vi "Begin Mouse.vi"(3 "Mouse IO":T1) -> (1 "Mouse IO out":T1)   [LabVIEW 2012]
uses:
  <vilib>/eio/EIONode/EIONode.xnode
  <vilib>/rvi/eio/common/nirviEmuTemplateMethod_errors.vi
  <vilib>/eio/EIOMethodNode/EIOMethodNode.xnode
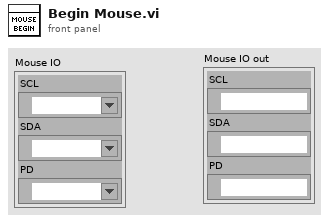
[diagram p1: front panel]
types:
  T1 = cluster{"SCL":refnum<k21>, "SDA":refnum<k21>, "PD":refnum<k21>}
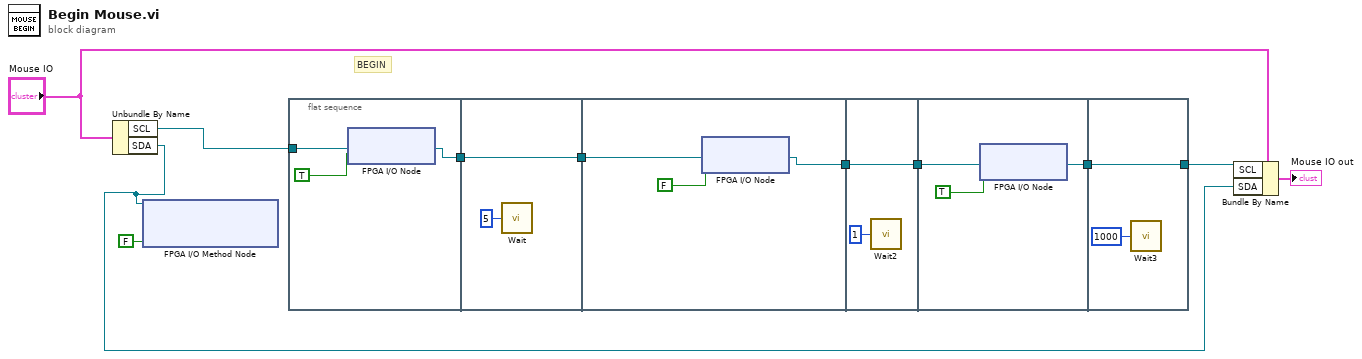
[diagram p0: block diagram]
diagram:
  # "BEGIN"
  n1 = Unbundle By Name("Mouse IO") -> ("SCL"=w7:refnum<k21>, "SDA"=w2:refnum<k21>)
  n2 = xnode "FPGA I/O Method Node"("FPGA I/O In"=w2, "Enable"=FALSE) -> ()  [unwired: 1 out]
  n3 = flat-sequence {
    tunnel: w7 -> [w14]
    tunnel: [w12] -> w11
    tunnel: [w16] -> w10
    tunnel: w11 -> [w16]
    tunnel: w10 -> [w18]
    tunnel: [w17] -> w9
    tunnel: [w21] -> w8
    tunnel: w9 -> [w21]
    tunnel: w8 -> [w23]
    tunnel: [w22] -> w5
    tunnel: [w25] -> w4
    tunnel: w5 -> [w25]
    frame #0 {
      n4 = xnode "FPGA I/O Node"("I/O Item"=TRUE, "FPGA I/O In"=w14) -> ("FPGA I/O Out"=w12:refnum<k21>)
    }
    frame #1 {
      n5 = call "Wait"("Count(uSec)"=u8 5) -> ()  [unwired: 1 out]
    }
    frame #2 {
      n6 = xnode "FPGA I/O Node"("I/O Item"=FALSE, "FPGA I/O In"=w18) -> ("FPGA I/O Out"=w17:refnum<k21>)
    }
    frame #3 {
      n7 = call "Wait2"("Count(uSec)"=u8 1) -> ()  [unwired: 1 out]
    }
    frame #4 {
      n8 = xnode "FPGA I/O Node"("I/O Item"=TRUE, "FPGA I/O In"=w23) -> ("FPGA I/O Out"=w22:refnum<k21>)
    }
    frame #5 {
      n9 = call "Wait3"("Count(mSec)"=u16 1000) -> ()  [unwired: 1 out]
    }
  }
  n10 = Bundle By Name(cluster="Mouse IO", "SCL"=w4, "SDA"=w2) -> (→"Mouse IO out":T1)
